vi "Pre Launch Init.vi"(11 "Test Caller Actor in":refnum<class "Test Caller Actor.lvclass">) -> (0 "error out":errorcluster, 3 "Test Caller Actor out":refnum<class "Test Caller Actor.lvclass">)   [LabVIEW 2023, in "Test Caller Actor.lvlib" / "Test Caller Actor.lvclass"]
doc: "(<B>Filename</B>: Actor Framework.lvlib:Actor.lvclass:Pre Launch Init.vi)\n\nDefines behavior that occurs after the Launch Nested Actor method is invoked but before the actor's Actor Core method begins running.\n\nBy default, this method does nothing. A descendant class may override it to define behavior."
uses:
  Test Caller Actor.lvclass
  Test Caller Actor.lvclass/Test Caller Actor.ctl
  Class Loader/Class Loader/Loading Progress.ctl
  Class Loader/Class Loader/Class Loader.lvclass
  <vilib>/ActorFramework/Actor/Actor.lvclass
  Load Complete Data.ctl
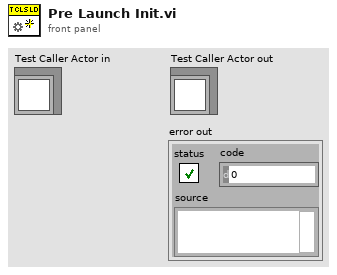
[diagram p1: front panel]
types:
  T1 = typedef "Test Caller Actor.lvlib/Test Caller Actor.lvclass/Load Complete Data.ctl" = cluster{"Load Complete":bool, "Class Names":string[]}
  T2 = typedef "Class Loader.lvlib/Class Loader.lvclass/Loading Progress.ctl" = dbl
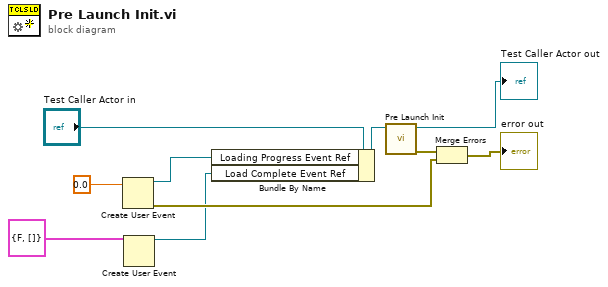
[diagram p0: block diagram]
diagram:
  n1 = Create User Event(user event datatype=T2 0.0 ("Loading Progress (%)")) -> (user event=w5:refnum<user-event>, error out=w3:errorcluster)  [unwired: 1 in]
  n2 = Create User Event(user event datatype=T1 {"Load Complete"=FALSE, "Class Names"=[]} ("Load Complete Data")) -> (user event=w2:refnum<user-event>)  [unwired: 1 in, 1 out]
  n3 = Bundle By Name(cluster="Test Caller Actor in", "Loading Progress Event Ref"=w5, "Load Complete Event Ref"=w2) -> (w6:refnum<class "Test Caller Actor.lvclass">)
  n4 = call-parent "Pre Launch Init.vi"("Actor in"=w6) -> ("error out"=w10:errorcluster, "Actor out"=→"Test Caller Actor out":refnum<class "Test Caller Actor.lvclass">)  [unwired: 9 in]
  n5 = Merge Errors(w10, w3) -> (→"error out":errorcluster)
